vi "Update Hardware Configuration File Error.vi"(8 "error in":errorcluster, 11 "configuration files ref in":T1 format="%.0x") -> (0 "error out":errorcluster, 3 "configuration files ref out":T1 format="%.0x")   [LabVIEW 2020, in "Ballard MIL-STD-1553 Scripting.lvlib"]
uses:
  Ballard MIL-STD-1553 Scripting.lvlib
  <vilib>/NI VeriStand/Custom Device API/Custom Device Item Ref.ctl
  Constants.vi
  <vilib>/NI VeriStand/Custom Device API/Custom Device API.lvlib
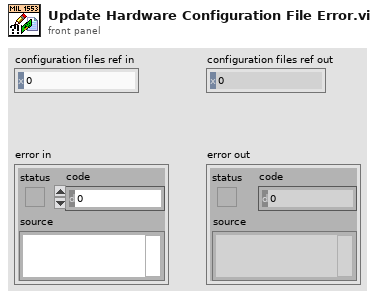
[diagram p1: front panel]
types:
  T1 = typedef "Custom Device API.lvlib/Custom Device Item Ref.ctl" = u64
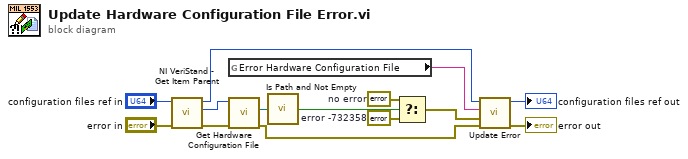
[diagram p0: block diagram]
diagram:
  w5 = errorcluster {"status"=FALSE, "code"=0, "source"=""}  # no error
  w6 = errorcluster {"status"=TRUE, "code"=-732358, "source"="hardware configuration file path must not be empty."}  # error -732358
  n1 = call <vilib>:"NI VeriStand - Get Item Parent.vi"("error in (no error)"="error in", "Item Ref in"="configuration files ref in") -> ("error out"=w10:errorcluster, "Parent Ref"=w9:T1, "Item Ref out"=w2:T1)  [unwired: 6 in, 1 out]
  n2 = global read "Constants.vi" "Error Hardware Configuration File"() -> (w1:string)
  n3 = call "Get Hardware Configuration File.vi"("error in"=w10, "Ballard MIL-STD 1553 custom device in"=w9) -> ("error out"=w4:errorcluster, "hardware configuration file"=w8:path)  [unwired: 6 in, 2 out]
  n4 = call <vilib>:"Is Path and Not Empty.vi"("path"=w8) -> ("Is Path and Not Empty?"=w7:bool)  [unwired: 4 in]
  n5 = Select(t=w5, s=w7, f=w6) -> (s? t:f=w3:errorcluster)
  n6 = call "Update Error.vi"("error in"=w4, "error to report"=w3, "error key"=w1, "section ref in"=w2) -> ("error out"=→"error out":errorcluster, "section ref out"=→"configuration files ref out":T1)  [unwired: 6 in]
